vi "Data_filtering_test.vi"() -> ()   [LabVIEW 2016]
panel:
  out "Waveform Graph":dbl[][](graph)
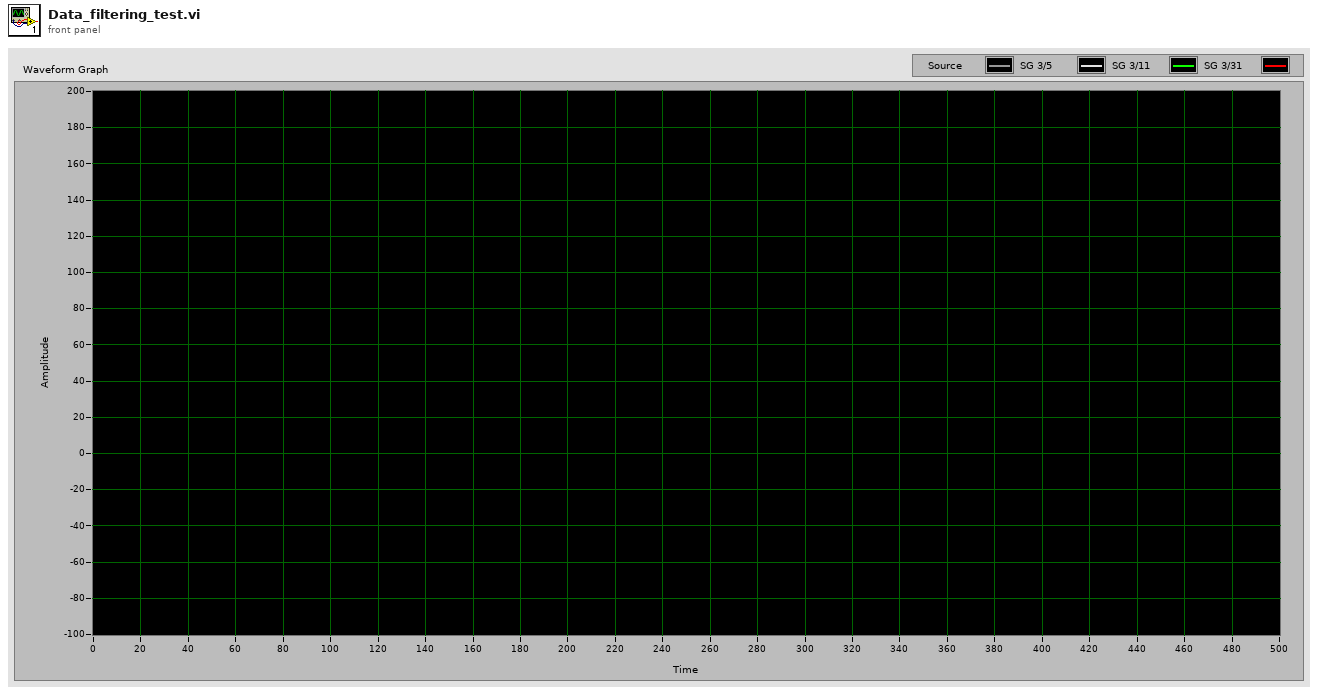
[diagram p1: front panel]
types:
  T1 = cluster{"0th order SG coefficients":dbl[], "1st order SG coefficients":dbl[]}
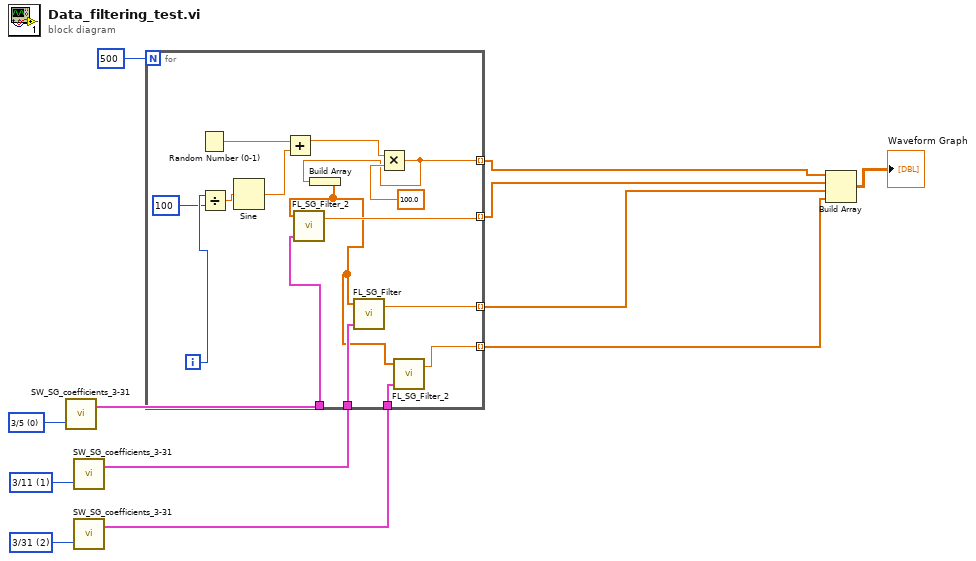
[diagram p0: block diagram]
diagram:
  w3 = u16 2 items=["3/5", "3/11", "3/31"] ("Select filter length")
  w6 = u16 1 items=["3/5", "3/11", "3/31"] ("Select filter length")
  w11 = u16 0 items=["3/5", "3/11", "3/31"] ("Select filter length")
  n1 = call "SW_SG_coefficients_3-31.vi"("Select filter length"=w11) -> ("SG coefficients"=w10:T1)  [unwired: 2 in]
  n2 = call "SW_SG_coefficients_3-31.vi"("Select filter length"=w6) -> ("SG coefficients"=w5:T1)  [unwired: 2 in]
  n3 = call "SW_SG_coefficients_3-31.vi"("Select filter length"=w3) -> ("SG coefficients"=w2:T1)  [unwired: 2 in]
  n4 = for {
    N: 500 -> [_]
    tunnel: [w20] -> w9 mode=indexing
    tunnel: w10 -> [w16]
    tunnel: [w17] -> w8 mode=indexing
    tunnel: w5 -> [w19]
    tunnel: [w18] -> w4 mode=indexing
    tunnel: w2 -> [w14]
    tunnel: [w13] -> w1 mode=indexing
    i -> [w23]
    n5 = Random Number (0-1)() -> (number: 0 to 1=w27:dbl)
    n6 = Divide(x=w23, y=100) -> (x/y=w24:dbl)
    n7 = Sine(x=w24) -> (sin(x)=w25:dbl)
    n8 = Add(x=w27, y=w25) -> (x+y=w21:dbl)
    n9 = Multiply(x=w21, y=100.0) -> (x*y=w20:dbl)
    n10 = Build Array(w20) -> (w15:dbl[])
    n11 = call "FL_SG_Filter_2.vi"("SG coefficients"=w16, "Input array of data"=w15) -> ("Filtered data, 0 order"=w17:dbl)  [unwired: 2 in]
    n12 = call "FL_SG_Filter.vi"("SG coefficients"=w19, "Input array of data"=w15) -> ("Filtered data, 0 order"=w18:dbl)  [unwired: 2 in]
    n13 = call "FL_SG_Filter_2.vi"("SG coefficients"=w14, "Input array of data"=w15) -> ("Filtered data, 0 order"=w13:dbl)  [unwired: 2 in]
  }
  n14 = Build Array(w9, w8, w4, w1) -> (→"Waveform Graph":dbl[][])
